vi "Bloco_leiturasSuper.vi"(10 "error in (no error)":errorcluster, 11 "reference":refnum<vi>) -> (0 "Status_Comunicacao":string, 1 "Led_status":bool, 2 "error out":errorcluster, 3 "reference out":refnum<vi>, 4 "Array_Tags/Config":string[](array[string]), 6 "todos_os_dados_ENTRADA":T1)   [LabVIEW 2019]
uses:
  \\SERVERPC\Server/padrao_todos_os_dados_ENTRADA.ctl
  \\SERVERPC\Server/padrao_ADAM_ENTRADA.ctl
  \\SERVERPC\Server/padrao_todos_os_dados_SAIDA.ctl
  \\SERVERPC\Server/padrao_UCM.004.EEL.0300_SAIDA.ctl
  \\SERVERPC\Server/padrao_UCM.004.EEL.0200_SAIDA.ctl
  \\SERVERPC\Server/padrao_INTERNO.ctl
  \\SERVERPC\Server/padrao_ADAM_SAIDA.ctl
  \\SERVERPC\Server/padrao_UCM.004.EEL.0300_ENTRADA.ctl
  \\SERVERPC\Server/padrao_UCM.004.EEL.0200_ENTRADA.ctl
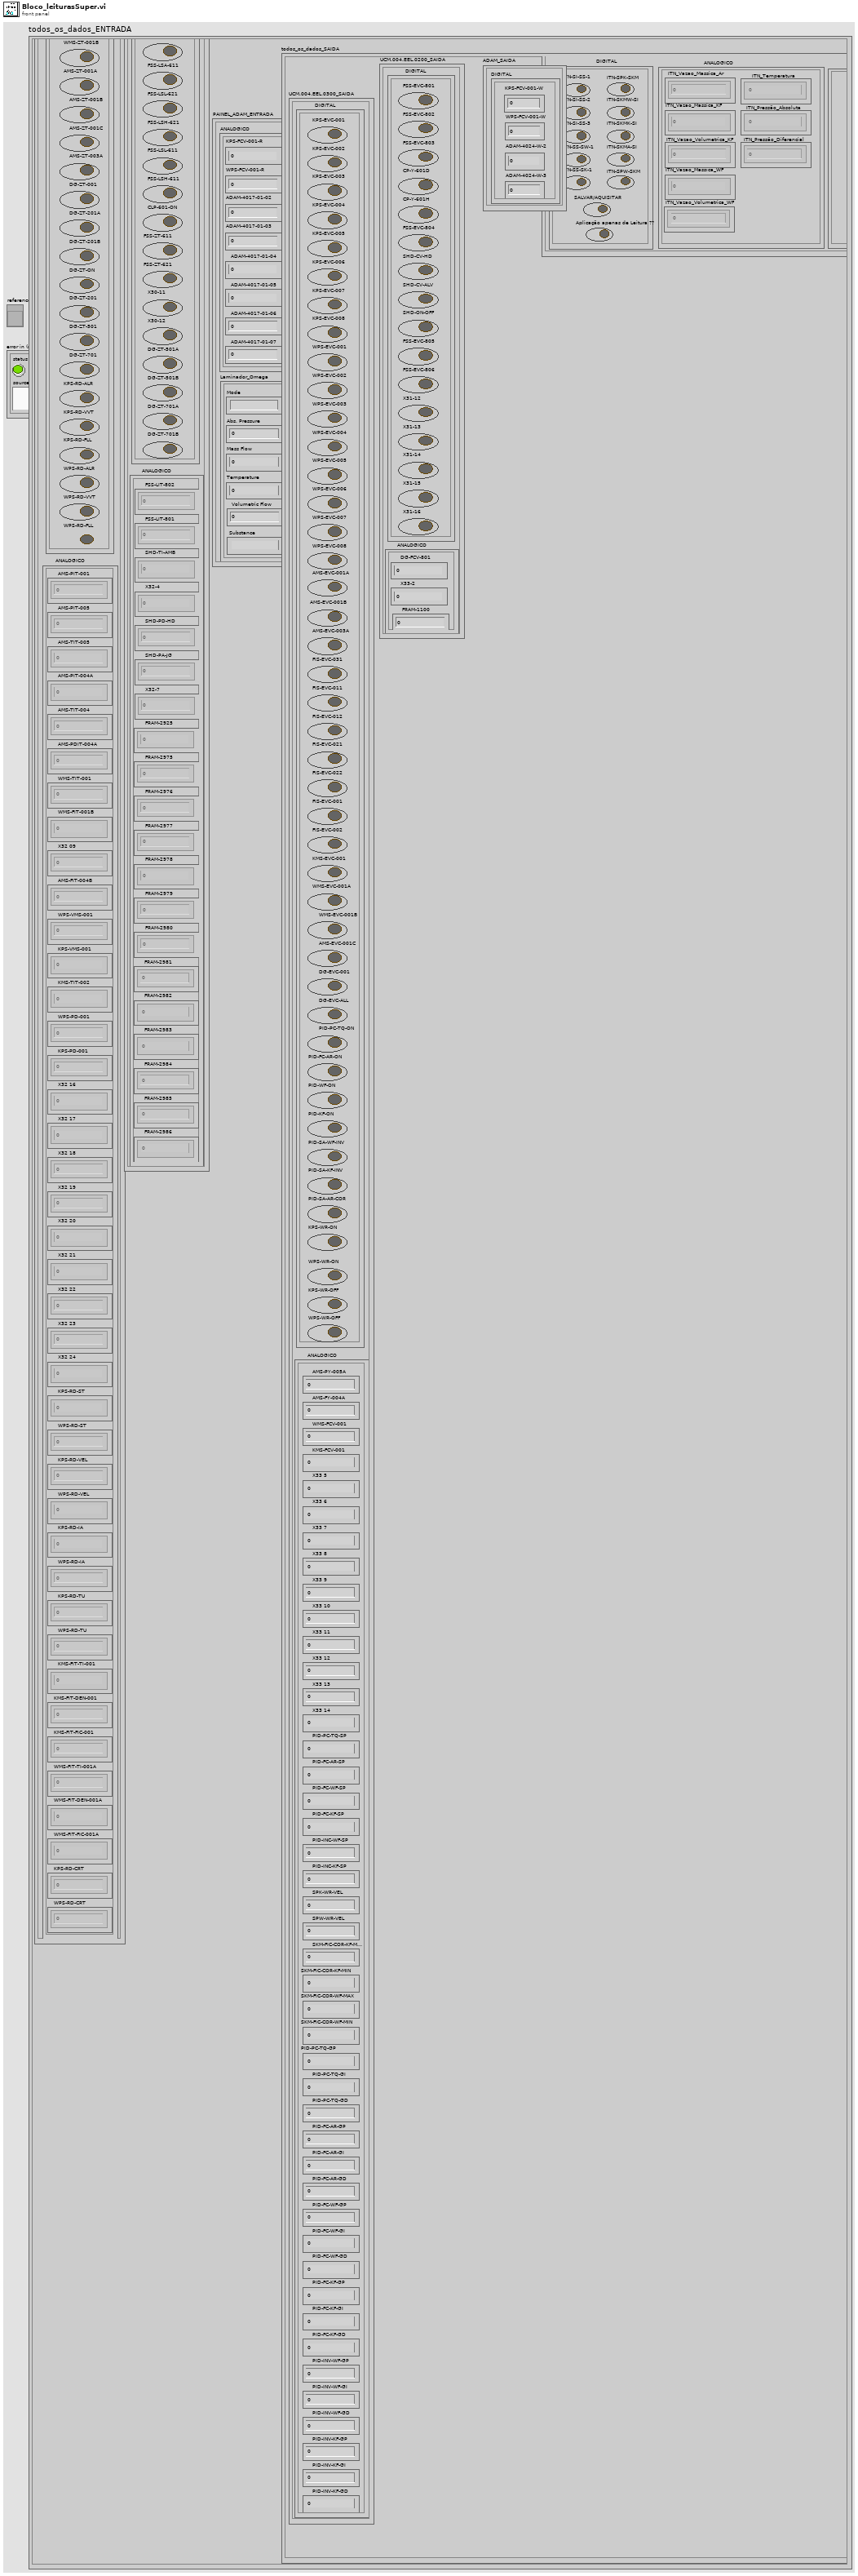
[diagram p1: front panel]
types:
  T1 = typedef "padrao_todos_os_dados_ENTRADA.ctl" = cluster{"PAINEL_ADAM_ENTRADA":T2, "todos_os_dados_SAIDA":T3, "UCM.004.EEL.0300_ENTRADA":T8, "UCM.004.EEL.0200_ENTRADA":T9}
  T2 = typedef "padrao_ADAM_ENTRADA.ctl" = cluster{"ANALOGICO":cluster{"KPS-FCV-001-R":dbl, "WPS-FCV-001-R":dbl, "ADAM-4017-01-02":dbl, "ADAM-4017-01-03":dbl, "ADAM-4017-01-04":dbl, "ADAM-4017-01-05":dbl, "ADAM-4017-01-06":dbl, "ADAM-4017-01-07":dbl}, "Laminador_Omega":cluster{"Mode ":string, "Abs. Pressure ":dbl, "Mass Flow":dbl, "Temperature":dbl, "Volumetric Flow":dbl, "Substance ":string}}
  T3 = typedef "padrao_todos_os_dados_SAIDA.ctl" = cluster{"UCM.004.EEL.0300_SAIDA":T4, "UCM.004.EEL.0200_SAIDA":T5, "INTERNO":T6, "ADAM_SAIDA":T7}
  T4 = typedef "padrao_UCM.004.EEL.0300_SAIDA.ctl" = cluster{"DIGITAL":cluster{"KPS-EVC-001":bool, "KPS-EVC-002":bool, "KPS-EVC-003":bool, "KPS-EVC-004":bool, "KPS-EVC-005":bool, "KPS-EVC-006":bool, "KPS-EVC-007":bool, "KPS-EVC-008":bool, "WPS-EVC-001":bool, "WPS-EVC-002":bool, "WPS-EVC-003":bool, "WPS-EVC-004":bool, "WPS-EVC-005":bool, "WPS-EVC-006":bool, "WPS-EVC-007":bool, "WPS-EVC-008":bool, "AMS-EVC-001B":bool, "AMS-EVC-003A":bool, "FIS-EVC-031":bool, "FIS-EVC-011":bool, "FIS-EVC-012":bool, "FIS-EVC-021":bool, "FIS-EVC-022":bool, "FIS-EVC-001":bool, "FIS-EVC-002":bool, "KMS-EVC-001":bool, "WMS-EVC-001A":bool, "WMS-EVC-001B":bool, "AMS-EVC-001C":bool, "DG-EVC-001":bool, "DG-EVC-ALL":bool, "PID-PC-TQ-ON":bool, "PID-FC-AR-ON":bool, "PID-WF-ON":bool, "PID-KF-ON":bool, "PID-SA-WF-INV":bool, "PID-SA-KF-INV":bool, "PID-SA-AR-COR":bool, "KPS-WR-ON":bool, "WPS-WR-ON":bool, "KPS-WR-OFF":bool, "WPS-WR-OFF":bool, "AMS-EVC-001A":bool}, "ANALOGICO":cluster{"AMS-PY-005A":i16, "AMS-FY-004A":i16, "WMS-FCV-001":i16, "KMS-FCV-001":i16, "X33 5":i16, "X33 6":i16, "X33 7":i16, "X33 8":i16, "X33 9":i16, "X33 10":i16, "X33 11":i16, "X33 12":i16, "X33 13":i16, "X33 14":i16, "PID-PC-TQ-SP":i16, "PID-FC-AR-SP":i16, "PID-FC-WF-SP":i16, "PID-FC-KF-SP":i16, "PID-INC-WF-SP":i16, "PID-INC-KF-SP":i16, "SPK-WR-VEL":i32, "SPW-WR-VEL":i32, "SKM-FIC-COR-KF-MAX":dbl, "SKM-FIC-COR-KF-MIN":dbl, "SKM-FIC-COR-WF-MAX":dbl, "SKM-FIC-COR-WF-MIN":dbl, "PID-PC-TQ-GP":dbl, "PID-PC-TQ-GI":dbl, "PID-PC-TQ-GD":dbl, "PID-FC-AR-GP":dbl, "PID-FC-AR-GI":dbl, "PID-FC-AR-GD":dbl, "PID-FC-WF-GP":dbl, "PID-FC-WF-GI":dbl, "PID-FC-WF-GD":dbl, "PID-FC-KF-GP":dbl, "PID-FC-KF-GI":dbl, "PID-FC-KF-GD":dbl, "PID-INV-WF-GP":dbl, "PID-INV-WF-GI":dbl, "PID-INV-WF-GD":dbl, "PID-INV-KF-GP":dbl, "PID-INV-KF-GI":dbl, "PID-INV-KF-GD":dbl}}
  T5 = typedef "padrao_UCM.004.EEL.0200_SAIDA.ctl" = cluster{"DIGITAL":cluster{"FSS-EVC-801":bool, "FSS-EVC-802":bool, "FSS-EVC-803":bool, "CP-Y-601D":bool, "CP-Y-601H":bool, "FSS-EVC-804":bool, "SHD-CV-HD":bool, "SHD-CV-ALV":bool, "SHD-ON-OFF":bool, "FSS-EVC-805":bool, "FSS-EVC-806":bool, "X31-12":bool, "X31-13":bool, "X31-14":bool, "X31-15":bool, "X31-16":bool}, "ANALOGICO":cluster{"DG-FCV-801":i16, "X33-2":i16, "FRAM-1100":i16}}
  T6 = typedef "padrao_INTERNO.ctl" = cluster{"DIGITAL":cluster{"ITN-SI-SS-1":bool, "ITN-SI-SS-2":bool, "ITN-SI-SS-3":bool, "ITN-SS-SW-1":bool, "ITN-SS-SK-1":bool, "ITN-SPW-SKM":bool, "ITN-SKMW-SI":bool, "ITN-SKMK-SI":bool, "ITN-SKMA-SI":bool, "ITN-SPK-SKM":bool, "Aplicação apenas de Leitura ??":bool, "SALVAR/AQUISITAR":bool}, "ANALOGICO":cluster{"ITN_Vazao_Massica_Ar":dbl[], "ITN_Vazao_Volumetrica_WF":dbl[], "ITN_Vazao_Massica_KF":dbl[], "ITN_Vazao_Massica_WF":dbl[], "ITN_Vazao_Volumetrica_KF":dbl[], "ITN_Temperatura":dbl[], "ITN_Pressão_Absoluta":dbl[], "ITN_Pressão_Diferencial":dbl[]}, "ALARMES-INTERNOS":cluster{"ALR-AMS-001A+B":bool, "ALR-AMS-001A+C":bool, "ALR-AMS-001B+C":bool, "ALR-AMS-001A+B+C":bool, "ALR-WMS-001A+B":bool}}
  T7 = typedef "padrao_ADAM_SAIDA.ctl" = cluster{"DIGITAL":cluster{"KPS-FCV-001-W":dbl, "WPS-FCV-001-W":dbl, "ADAM-4024-W-2":dbl, "ADAM-4024-W-3":dbl}}
  T8 = typedef "padrao_UCM.004.EEL.0300_ENTRADA.ctl" = cluster{"DIGITAL":cluster{"ADAM-ON":bool, "CLP-ON":bool, "KMS-ZT-001":bool, "WMS-ZT-001A":bool, "WMS-ZT-001B":bool, "AMS-ZT-001A":bool, "AMS-ZT-001B":bool, "AMS-ZT-001C":bool, "AMS-ZT-003A":bool, "DG-ZT-001":bool, "DG-ZT-201A":bool, "DG-ZT-201B":bool, "DG-ZT-ON":bool, "DG-ZT-201":bool, "DG-ZT-501":bool, "DG-ZT-701":bool, "KPS-RD-ALR":bool, "KPS-RD-VVT":bool, "KPS-RD-FLL":bool, "WPS-RD-ALR":bool, "WPS-RD-VVT":bool, "WPS-RD-FLL":bool}, "ANALOGICO":cluster{"AMS-PIT-001":dbl[], "AMS-PIT-005":dbl[], "AMS-TIT-005":dbl[], "AMS-PIT-004A":dbl[], "AMS-TIT-004":dbl[], "AMS-PDIT-004A":dbl[], "WMS-TIT-001":dbl[], "WMS-FIT-001B":dbl[], "X32 09":dbl[], "AMS-FIT-004B":dbl[], "WPS-VMS-001":dbl[], "KPS-VMS-001":dbl[], "KMS-TIT-002":dbl[], "WPS-PD-001":dbl[], "KPS-PD-001":dbl[], "X32 16 ":dbl[], "X32 17":dbl[], "X32 18":dbl[], "X32 19":dbl[], "X32 20":dbl[], "X32 21":dbl[], "X32 22":dbl[], "X32 23":dbl[], "X32 24":dbl[], "KPS-RD-ST":dbl[], "WPS-RD-ST":dbl[], "KPS-RD-VEL":dbl[], "WPS-RD-VEL":dbl[], "KPS-RD-IA":dbl[], "WPS-RD-IA":dbl[], "KPS-RD-TU":dbl[], "WPS-RD-TU":dbl[], "KMS-FIT-TI-001":dbl[], "KMS-FIT-DEN-001":dbl[], "KMS-FIT-FIC-001":dbl[], "WMS-FIT-TI-001A":dbl[], "WMS-FIT-DEN-001A":dbl[], "KPS-RD-CRT":dbl[], "WPS-RD-CRT":dbl[], "WMS-FIT-FIC-001A":dbl[]}}
  T9 = typedef "padrao_UCM.004.EEL.0200_ENTRADA.ctl" = cluster{"DIGITAL":cluster{"FSS-LSA-801":bool, "FSS-LSA-621":bool, "FSS-LSA-611":bool, "FSS-LSL-621":bool, "FSS-LSH-621":bool, "FSS-LSL-611":bool, "FSS-LSH-611":bool, "CLP-601-ON":bool, "FSS-ZT-611":bool, "FSS-ZT-621":bool, "X30-11":bool, "X30-12":bool, "DG-ZT-501A":bool, "DG-ZT-501B":bool, "DG-ZT-701A":bool, "DG-ZT-701B":bool}, "ANALOGICO":cluster{"FSS-LIT-802":dbl[], "FSS-LIT-801":dbl[], "SHD-TI-AMB":dbl[], "X32-4":dbl[], "SHD-PD-HD":dbl[], "SHD-PA-JG":dbl[], "X32-7":dbl[], "FRAM-2925":dbl[], "FRAM-2975":dbl[], "FRAM-2976":dbl[], "FRAM-2977":dbl[], "FRAM-2978":dbl[], "FRAM-2979":dbl[], "FRAM-2980":dbl[], "FRAM-2981":dbl[], "FRAM-2982":dbl[], "FRAM-2983":dbl[], "FRAM-2984":dbl[], "FRAM-2985":dbl[], "FRAM-2986":dbl[], "FRAM-2987":dbl[]}}
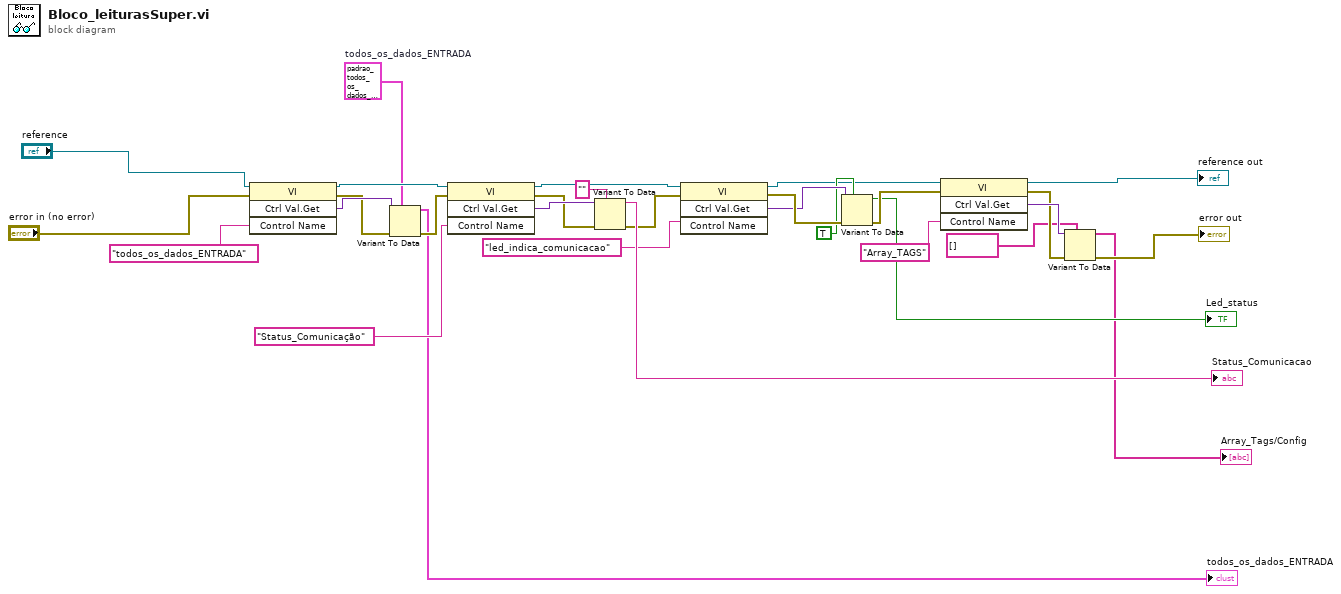
[diagram p0: block diagram]
diagram:
  w2 = T1 {"PAINEL_ADAM_ENTRADA"={"ANALOGICO"={"KPS-FCV-001-R"=0.0, "WPS-FCV-001-R"=0.0, "ADAM-4017-01-02"=0.0, "ADAM-4017-01-03"=0.0, "ADAM-4017-01-04"=0.0, "ADAM-4017-01-05"=0.0, "ADAM-4017-01-06"=0.0, "ADAM-4017-01-07"=0.0}, "Laminador_Omega"={"Mode "="", "Abs. Pressure "=0.0, "Mass Flow"=0.0, "Temperature"=0.0, "Volumetric Flow"=0.0, "Substance "=""}}, "todos_os_dados_SAIDA"={"UCM.004.EEL.0300_SAIDA"={"DIGITAL"={"KPS-EVC-001"=FALSE, "KPS-EVC-002"=FALSE, "KPS-EVC-003"=FALSE, "KPS-EVC-004"=FALSE, "KPS-EVC-005"=FALSE, "KPS-EVC-006"=FALSE, "KPS-EVC-007"=FALSE, "KPS-EVC-008"=FALSE, "WPS-EVC-001"=FALSE, "WPS-EVC-002"=FALSE, "WPS-EVC-003"=FALSE, "WPS-EVC-004"=FALSE, "WPS-EVC-005"=FALSE, "WPS-EVC-006"=FALSE, "WPS-EVC-007"=FALSE, "WPS-EVC-008"=FALSE, "AMS-EVC-001B"=FALSE, "AMS-EVC-003A"=FALSE, "FIS-EVC-031"=FALSE, "FIS-EVC-011"=FALSE, "FIS-EVC-012"=FALSE, "FIS-EVC-021"=FALSE, "FIS-EVC-022"=FALSE, "FIS-EVC-001"=FALSE, "FIS-EVC-002"=FALSE, "KMS-EVC-001"=FALSE, "WMS-EVC-001A"=FALSE, "WMS-EVC-001B"=FALSE, "AMS-EVC-001C"=FALSE, "DG-EVC-001"=FALSE, "DG-EVC-ALL"=FALSE, "PID-PC-TQ-ON"=FALSE, "PID-FC-AR-ON"=FALSE, "PID-WF-ON"=FALSE, "PID-KF-ON"=FALSE, "PID-SA-WF-INV"=FALSE, "PID-SA-KF-INV"=FALSE, "PID-SA-AR-COR"=FALSE, "KPS-WR-ON"=FALSE, "WPS-WR-ON"=FALSE, "KPS-WR-OFF"=FALSE, "WPS-WR-OFF"=FALSE, "AMS-EVC-001A"=FALSE}, "ANALOGICO"={"AMS-PY-005A"=0, "AMS-FY-004A"=0, "WMS-FCV-001"=0, "KMS-FCV-001"=0, "X33 5"=0, "X33 6"=0, "X33 7"=0, "X33 8"=0, "X33 9"=0, "X33 10"=0, "X33 11"=0, "X33 12"=0, "X33 13"=0, "X33 14"=0, "PID-PC-TQ-SP"=0, "PID-FC-AR-SP"=0, "PID-FC-WF-SP"=0, "PID-FC-KF-SP"=0, "PID-INC-WF-SP"=0, "PID-INC-KF-SP"=0, "SPK-WR-VEL"=0, "SPW-WR-VEL"=0, "SKM-FIC-COR-KF-MAX"=0.0, "SKM-FIC-COR-KF-MIN"=0.0, "SKM-FIC-COR-WF-MAX"=0.0, "SKM-FIC-COR-WF-MIN"=0.0, "PID-PC-TQ-GP"=0.0, "PID-PC-TQ-GI"=0.0, "PID-PC-TQ-GD"=0.0, "PID-FC-AR-GP"=0.0, "PID-FC-AR-GI"=0.0, "PID-FC-AR-GD"=0.0, "PID-FC-WF-GP"=0.0, "PID-FC-WF-GI"=0.0, "PID-FC-WF-GD"=0.0, "PID-FC-KF-GP"=0.0, "PID-FC-KF-GI"=0.0, "PID-FC-KF-GD"=0.0, "PID-INV-WF-GP"=0.0, "PID-INV-WF-GI"=0.0, "PID-INV-WF-GD"=0.0, "PID-INV-KF-GP"=0.0, "PID-INV-KF-GI"=0.0, "PID-INV-KF-GD"=0.0}}, "UCM.004.EEL.0200_SAIDA"={"DIGITAL"={"FSS-EVC-801"=FALSE, "FSS-EVC-802"=FALSE, "FSS-EVC-803"=FALSE, "CP-Y-601D"=FALSE, "CP-Y-601H"=FALSE, "FSS-EVC-804"=FALSE, "SHD-CV-HD"=FALSE, "SHD-CV-ALV"=FALSE, "SHD-ON-OFF"=FALSE, "FSS-EVC-805"=FALSE, "FSS-EVC-806"=FALSE, "X31-12"=FALSE, "X31-13"=FALSE, "X31-14"=FALSE, "X31-15"=FALSE, "X31-16"=FALSE}, "ANALOGICO"={"DG-FCV-801"=0, "X33-2"=0, "FRAM-1100"=0}}, "INTERNO"={"DIGITAL"={"ITN-SI-SS-1"=FALSE, "ITN-SI-SS-2"=FALSE, "ITN-SI-SS-3"=FALSE, "ITN-SS-SW-1"=FALSE, "ITN-SS-SK-1"=FALSE, "ITN-SPW-SKM"=FALSE, "ITN-SKMW-SI"=FALSE, "ITN-SKMK-SI"=FALSE, "ITN-SKMA-SI"=FALSE, "ITN-SPK-SKM"=FALSE, "Aplicação apenas de Leitura ??"=FALSE, "SALVAR/AQUISITAR"=FALSE}, "ANALOGICO"={"ITN_Vazao_Massica_Ar"=[], "ITN_Vazao_Volumetrica_WF"=[], "ITN_Vazao_Massica_KF"=[], "ITN_Vazao_Massica_WF"=[], "ITN_Vazao_Volumetrica_KF"=[], "ITN_Temperatura"=[], "ITN_Pressão_Absoluta"=[], "ITN_Pressão_Diferencial"=[]}, "ALARMES-INTERNOS"={"ALR-AMS-001A+B"=FALSE, "ALR-AMS-001A+C"=FALSE, "ALR-AMS-001B+C"=FALSE, "ALR-AMS-001A+B+C"=FALSE, "ALR-WMS-001A+B"=FALSE}}, "ADAM_SAIDA"={"DIGITAL"={"KPS-FCV-001-W"=0.0, "WPS-FCV-001-W"=0.0, "ADAM-4024-W-2"=0.0, "ADAM-4024-W-3"=0.0}}}, "UCM.004.EEL.0300_ENTRADA"={"DIGITAL"={"ADAM-ON"=FALSE, "CLP-ON"=FALSE, "KMS-ZT-001"=FALSE, "WMS-ZT-001A"=FALSE, "WMS-ZT-001B"=FALSE, "AMS-ZT-001A"=FALSE, "AMS-ZT-001B"=FALSE, "AMS-ZT-001C"=FALSE, "AMS-ZT-003A"=FALSE, "DG-ZT-001"=FALSE, "DG-ZT-201A"=FALSE, "DG-ZT-201B"=FALSE, "DG-ZT-ON"=FALSE, "DG-ZT-201"=FALSE, "DG-ZT-501"=FALSE, "DG-ZT-701"=FALSE, "KPS-RD-ALR"=FALSE, "KPS-RD-VVT"=FALSE, "KPS-RD-FLL"=FALSE, "WPS-RD-ALR"=FALSE, "WPS-RD-VVT"=FALSE, "WPS-RD-FLL"=FALSE}, "ANALOGICO"={"AMS-PIT-001"=[], "AMS-PIT-005"=[], "AMS-TIT-005"=[], "AMS-PIT-004A"=[], "AMS-TIT-004"=[], "AMS-PDIT-004A"=[], "WMS-TIT-001"=[], "WMS-FIT-001B"=[], "X32 09"=[], "AMS-FIT-004B"=[], "WPS-VMS-001"=[], "KPS-VMS-001"=[], "KMS-TIT-002"=[], "WPS-PD-001"=[], "KPS-PD-001"=[], "X32 16 "=[], "X32 17"=[], "X32 18"=[], "X32 19"=[], "X32 20"=[], "X32 21"=[], "X32 22"=[], "X32 23"=[], "X32 24"=[], "KPS-RD-ST"=[], "WPS-RD-ST"=[], "KPS-RD-VEL"=[], "WPS-RD-VEL"=[], "KPS-RD-IA"=[], "WPS-RD-IA"=[], "KPS-RD-TU"=[], "WPS-RD-TU"=[], "KMS-FIT-TI-001"=[], "KMS-FIT-DEN-001"=[], "KMS-FIT-FIC-001"=[], "WMS-FIT-TI-001A"=[], "WMS-FIT-DEN-001A"=[], "KPS-RD-CRT"=[], "WPS-RD-CRT"=[], "WMS-FIT-FIC-001A"=[]}}, "UCM.004.EEL.0200_ENTRADA"={"DIGITAL"={"FSS-LSA-801"=FALSE, "FSS-LSA-621"=FALSE, "FSS-LSA-611"=FALSE, "FSS-LSL-621"=FALSE, "FSS-LSH-621"=FALSE, "FSS-LSL-611"=FALSE, "FSS-LSH-611"=FALSE, "CLP-601-ON"=FALSE, "FSS-ZT-611"=FALSE, "FSS-ZT-621"=FALSE, "X30-11"=FALSE, "X30-12"=FALSE, "DG-ZT-501A"=FALSE, "DG-ZT-501B"=FALSE, "DG-ZT-701A"=FALSE, "DG-ZT-701B"=FALSE}, "ANALOGICO"={"FSS-LIT-802"=[], "FSS-LIT-801"=[], "SHD-TI-AMB"=[], "X32-4"=[], "SHD-PD-HD"=[], "SHD-PA-JG"=[], "X32-7"=[], "FRAM-2925"=[], "FRAM-2975"=[], "FRAM-2976"=[], "FRAM-2977"=[], "FRAM-2978"=[], "FRAM-2979"=[], "FRAM-2980"=[], "FRAM-2981"=[], "FRAM-2982"=[], "FRAM-2983"=[], "FRAM-2984"=[], "FRAM-2985"=[], "FRAM-2986"=[], "FRAM-2987"=[]}}}  # todos_os_dados_ENTRADA
  n1 = invoke class="VI" method="Ctrl Val.Get"(reference="reference", error in="error in (no error)", "Control Name"="todos_os_dados_ENTRADA") -> (reference out=w27:refnum<vi>, error out=w28:errorcluster, "Get Control Value Variant"=w29:variant)  [unwired: 1 in, 1 out]
  n2 = Variant To Data(error in=w28, type=w2, Variant=w29) -> (data=→"todos_os_dados_ENTRADA":T1, error out=w26:errorcluster)
  n3 = invoke class="VI" method="Ctrl Val.Get"(reference=w27, error in=w26, "Control Name"="Status_Comunicação") -> (reference out=w16:refnum<vi>, error out=w21:errorcluster, "Get Control Value Variant"=w24:variant)  [unwired: 1 in, 1 out]
  n4 = Variant To Data(error in=w21, type="", Variant=w24) -> (data=→"Status_Comunicacao":string, error out=w17:errorcluster)
  n5 = invoke class="VI" method="Ctrl Val.Get"(reference=w16, error in=w17, "Control Name"="led_indica_comunicacao") -> (reference out=w14:refnum<vi>, error out=w20:errorcluster, "Get Control Value Variant"=w19:variant)  [unwired: 1 in, 1 out]
  n6 = Variant To Data(error in=w20, type=TRUE, Variant=w19) -> (data=→"Led_status":bool, error out=w13:errorcluster)
  n7 = invoke class="VI" method="Ctrl Val.Get"(reference=w14, error in=w13, "Control Name"="Array_TAGS") -> (reference out=→"reference out":refnum<vi>, error out=w10:errorcluster, "Get Control Value Variant"=w11:variant)  [unwired: 1 in, 1 out]
  n8 = Variant To Data(error in=w10, type=string[] [] ("Array - String"), Variant=w11) -> (data=→"Array_Tags/Config":string[], error out=→"error out":errorcluster)
